vi "OAT Polar Autoscale as Needed.vi"(1 "polar attributes":T1={"maximum"=1.0, "minimum"=0.0, "clip to min"=FALSE, "log"=FALSE, "grid color"=0, "plot color"=0, "fmt and prec"={"format"=enum."Decimal", "precision"=2}, "visible section"=8} {"minimum" format="%.2f"; "maximum" format="%.2f"}, 2 "magnitudes (even angular)":dbl[](array[numeric]) format="%.2f") -> (0 "polar attributes":T1={"maximum"=1.0, "minimum"=0.0, "clip to min"=FALSE, "log"=FALSE, "grid color"=0, "plot color"=0, "fmt and prec"={"format"=enum."Decimal", "precision"=2}, "visible section"=8} {"minimum" format="%.2e"; "maximum" format="%.2e"})   [LabVIEW 2017]
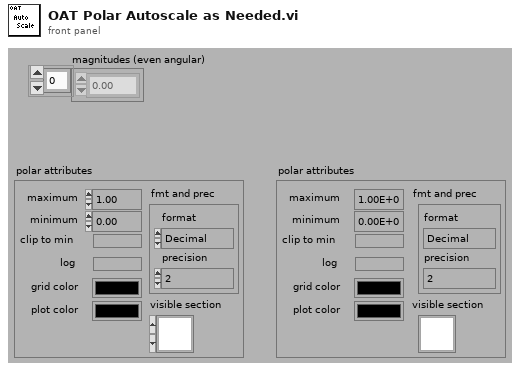
[diagram p1: front panel]
types:
  T1 = cluster{"maximum":dbl, "minimum":dbl, "clip to min":bool, "log":bool, "grid color":u32, "plot color":u32, "fmt and prec":cluster{"format":enum8{"Decimal", "Scientific", "Engineering", "Binary", "Octal", "Hex"}, "precision":u8}, "visible section":u16}
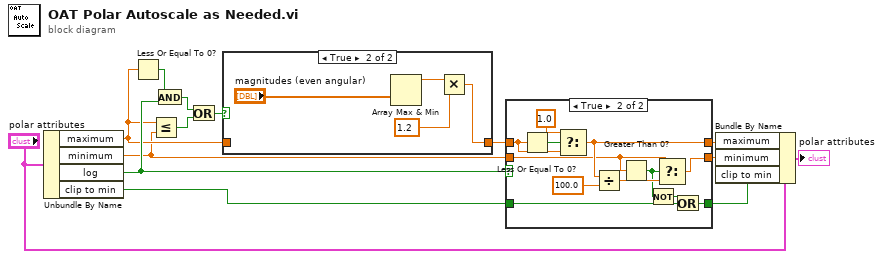
[diagram p0: block diagram]
diagram:
  n1 = Unbundle By Name("polar attributes") -> ("maximum"=w5:dbl, "minimum"=w4:dbl, "log"=w7:bool, "clip to min"=w1:bool)
  n2 = Less Or Equal To 0?(x=w5) -> (x <= 0?=w6:bool)
  n3 = Less Or Equal?(x=w5, y=w4) -> (x <= y?=w9:bool)
  n4 = And(x=w6, y=w7) -> (x .and. y?=w10:bool)
  n5 = Or(x=w10, y=w9) -> (x .or. y?=w8:bool)
  n6 = case shown="True" w8 {
    tunnel: w5 -> [w15 _]
    tunnel: [w15 w17] -> w11
    frame False {
    }
    frame True {
      n7 = Array Max & Min(array="magnitudes (even angular)") -> (max value=w19:dbl)  [unwired: 3 out]
      n8 = Multiply(x=w19, y=1.2 ("t")) -> (x*y=w17:dbl)
    }
  }
  n9 = case shown="True" w7 {
    tunnel: w4 -> [w22 w29]
    tunnel: [w22 w28] -> w12
    tunnel: w11 -> [w21 w32]
    tunnel: [w21 w30] -> w3
    tunnel: [w20 w24] -> w2
    tunnel: w1 -> [w20 w25]
    frame False {
    }
    frame True {
      n10 = Less Or Equal To 0?(x=w32) -> (x <= 0?=w33:bool)
      n11 = Select(t=1.0, s=w33, f=w32) -> (s? t:f=w30:dbl)
      n12 = Divide(x=w30, y=100.0) -> (x/y=w27:dbl)
      n13 = Greater Than 0?(x=w29) -> (x > 0?=w26:bool)
      n14 = Not(x=w26) -> (.not. x?=w23:bool)
      n15 = Select(t=w29, s=w26, f=w27) -> (s? t:f=w28:dbl)
      n16 = Or(x=w23, y=w25) -> (x .or. y?=w24:bool)
    }
  }
  n17 = Bundle By Name(cluster="polar attributes", "maximum"=w3, "minimum"=w12, "clip to min"=w2) -> (→"polar attributes":T1)
